vi "Open Block Diagram.vi"(8 "error in (no error)":errorcluster, 11 "VI Path":path) -> (0 "error out":errorcluster, 3 "VI Path Out":path)   [LabVIEW 2016, in "SLL Class DVR API Generator.lvlib"]
uses:
  SLL Class DVR API Generator.lvlib
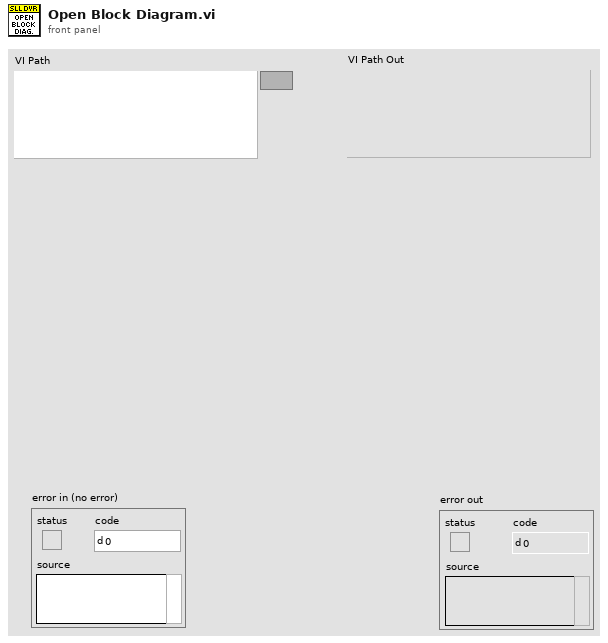
[diagram p1: front panel]
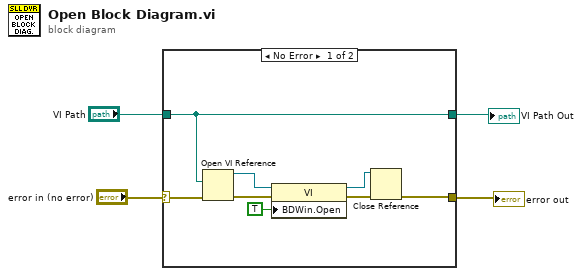
[diagram p0: block diagram]
diagram:
  n1 = case shown="No Error" "error in (no error)" {
    selector: "error in (no error)" -> [w12 w14]
    tunnel: [w6 w14] -> w3
    tunnel: "VI Path" -> [w5 w13]
    tunnel: [w5 w13] -> w1
    frame No Error {
      n2 = Open VI Reference(vi path=w5, error in (no error)=w12) -> (vi reference=w10:refnum<vi>, error out=w11:errorcluster)  [unwired: 4 in]
      n3 = property class="VI"(reference=w10, error in=w11, "BDWin.Open"=TRUE ("Block Diagram Window:Open")) -> (reference out=w7:refnum<vi>, error out=w8:errorcluster)
      n4 = Close Reference(reference=w7, error in (no error)=w8) -> (error out=w6:errorcluster)
    }
    frame Error {
    }
  }
  "error out" <- w3
  "VI Path Out" <- w1
